vi "Get Test Method Type.vi"(10 "Failure String":string) -> (2 "method type":enum16{"setUp", "testMethod", "tearDown"}(ring))   [LabVIEW 2011, in "GraphicalTestRunner.lvlib"]
uses:
  GraphicalTestRunner.lvlib
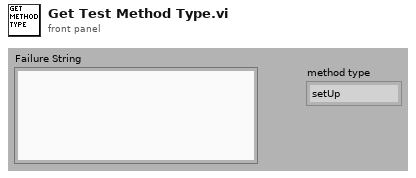
[diagram p1: front panel]
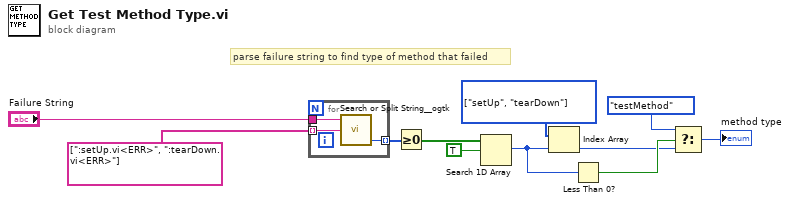
[diagram p0: block diagram]
diagram:
  w8 = enum16{"setUp", "testMethod", "tearDown"}[] [enum."setUp", enum."tearDown"] items=["setUp", "testMethod", "tearDown"]
  # "parse failure string to find type of method that failed"
  n1 = for {
    tunnel: "Failure String" -> [w14]
    tunnel: string[] [":setUp.vi<ERR>", ":tearDown.vi<ERR>"] -> [w13] mode=indexing
    tunnel: [w12] -> w11 mode=indexing
    n2 = call <userlib>:"Search or Split String__ogtk.vi"("search string/char (-)"=w13, "string"=w14) -> ("offset after match"=w12:i32)  [unwired: 1 in, 2 out]
  }
  n3 = Greater Or Equal To 0?(x=w11) -> (x >= 0?=w7:bool[])
  n4 = Search 1D Array(1D array=w7, element=TRUE) -> (index of element=w6:i32)  [unwired: 1 in]
  n5 = Index Array(array=w8, index=w6) -> (element=w3:enum16{"setUp", "testMethod", "tearDown"})
  n6 = Less Than 0?(x=w6) -> (x < 0?=w5:bool)
  n7 = Select(t=enum16{"setUp", "testMethod", "tearDown"}."testMethod" ("Method (testMethod)"), s=w5, f=w3) -> (s? t:f=→"method type":enum16{"setUp", "testMethod", "tearDown"})
